vi "Update Custom Device XML.vi"(5 "Template Folder":path, 8 "error in":errorcluster, 10 "Custom Device Name":string, 11 "CDEW_MetaDataObj in":refnum<class "NIVS_CDEW_MetaDataObj.lvclass">) -> (0 "error out":errorcluster, 3 "Custom Device XML Path":path)   [LabVIEW 2026, in "NIVS_CDEW_MetaDataObj.lvclass"]
uses:
  NIVS_CDEW_MetaDataObj.lvclass
  NIVS_CDEW_MetaDataObj.lvclass/NIVS_CDEW_MetaDataObj.ctl
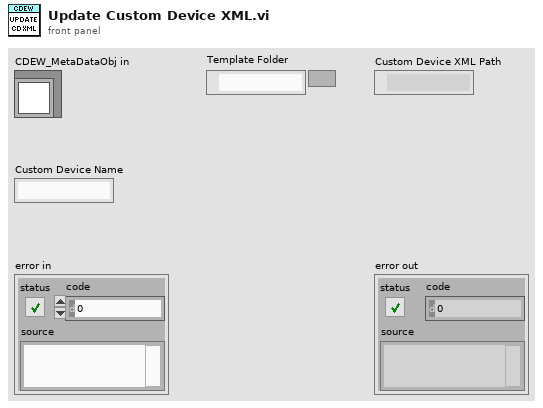
[diagram p1: front panel]
types:
  T1 = typedef "NIVS_CDEW_MetaDataObj.lvclass/Execution Modes.ctl" = enum16{"Inline HW Interface (Inline-Async API)", "Inline HW Interface", "Inline Timing and Sync"}
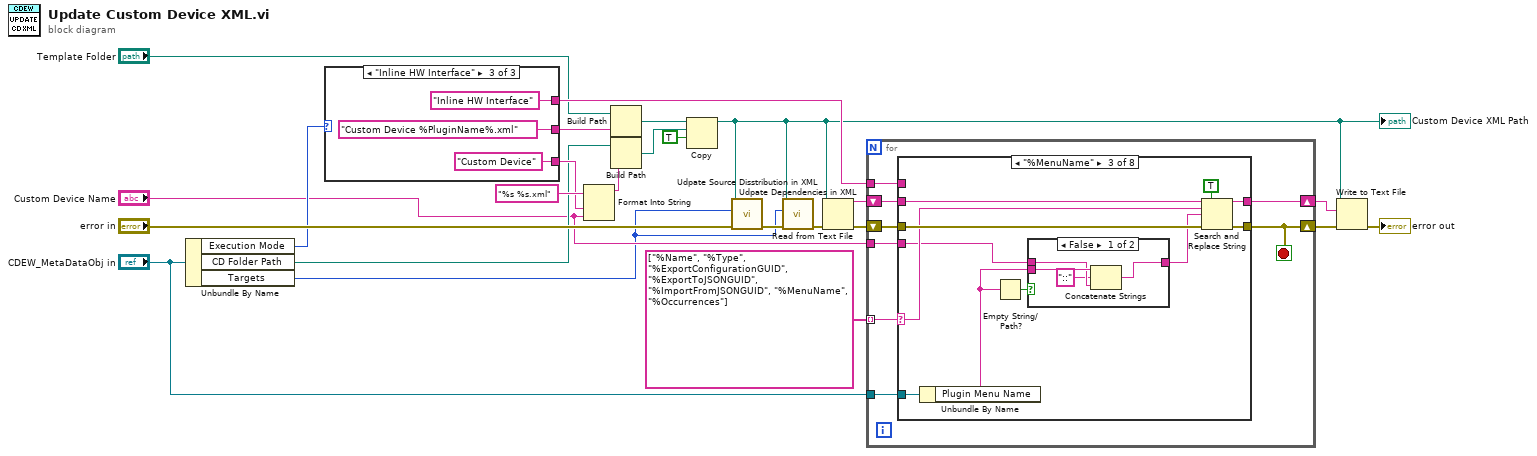
[diagram p0: block diagram]
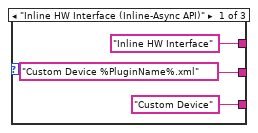
[diagram p2: hidden frame]
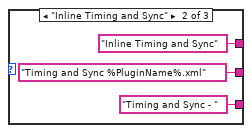
[diagram p3: hidden frame]
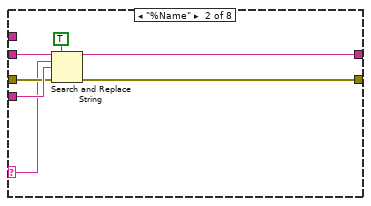
[diagram p5: hidden frame]
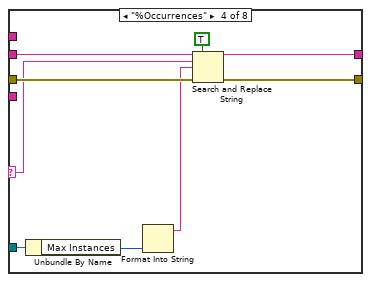
[diagram p7: hidden frame]
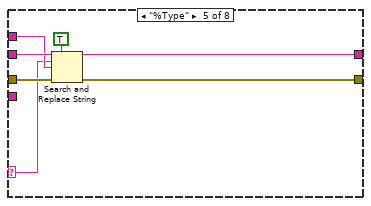
[diagram p8: hidden frame]
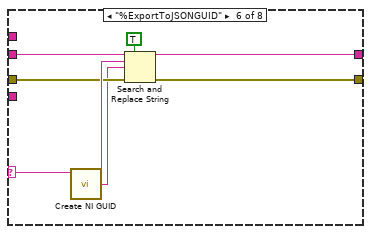
[diagram p9: hidden frame]
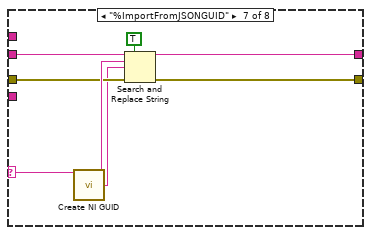
[diagram p10: hidden frame]
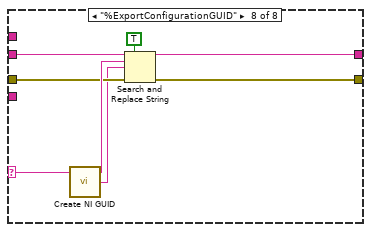
[diagram p11: hidden frame]
diagram:
  n1 = Unbundle By Name("CDEW_MetaDataObj in") -> ("Execution Mode"=w7:T1, "CD Folder Path"=w8:path, "Targets"=w1:enum16{"Linux_x64", "Windows", "Both"})
  n2 = case shown="\"Inline HW Interface\"" w7 {
    tunnel: ["Inline HW Interface" ("Plugin Type") "Inline Timing and Sync" ("Plugin Type") "Inline HW Interface" ("Plugin Type")] -> w18
    tunnel: ["Custom Device %PluginName%.xml" "Timing and Sync %PluginName%.xml" "Custom Device %PluginName%.xml"] -> w16
    tunnel: ["Custom Device" ("Plugin Type") "Timing and Sync - " ("Plugin Type") "Custom Device" ("Plugin Type")] -> w11
    frame "Inline HW Interface (Inline-Async API)" {
    }
    frame "Inline Timing and Sync" {
    }
    frame "Inline HW Interface" {
    }
  }
  n3 = Format Into String(format string="%s %s.xml", w11, "Custom Device Name") -> (resulting string=w10:string)  [unwired: 2 in, 1 out]
  n4 = Build Path(base path="Template Folder", name or relative path=w16) -> (appended path=w15:path)
  n5 = Build Path(base path=w8, name or relative path=w10) -> (appended path=w14:path)
  n6 = Copy(9:TRUE ("overwrite (F)"), 10:w14, 11:w15) -> (3:w2:path)  [unwired: 2 in, 2 out]
  "Custom Device XML Path" <- w2
  n7 = call "Udpate Source Disstribution in XML.vi"("error in"="error in", "Targets"=w1, "XML path"=w2) -> ("error out"=w4:errorcluster)  [unwired: 8 in]
  n8 = call "Udpate Dependencies in XML.vi"("error in"=w4, "Targets"=w1, "XML path"=w2) -> ("error out"=w3:errorcluster)  [unwired: 8 in]
  n9 = Read from Text File(file (use dialog)=w2, error in=w3) -> (text=w23:string, error out=w20:errorcluster)  [unwired: 2 in, 2 out]
  n10 = for {
    tunnel: string[] ["%Name", "%Type", "%ExportConfigurationGUID", "%ExportToJSONGUID", "%ImportFromJSONGUID", "%MenuName", "%Occurrences"] -> [w39] mode=indexing
    shift-right: [w40] -> w22
    shift-left: w23 -> [w41]
    tunnel: "Custom Device Name" -> [w38]
    tunnel: w18 -> [w37]
    shift-right: [w35] -> w19
    shift-left: w20 -> [w36]
    tunnel: "CDEW_MetaDataObj in" -> [w34]
    stop <- w35 stop-if-true
    n11 = case shown="\"%MenuName\"" w39 {
      selector: w39 -> [_ w44 w56 w70 w77 w86 w93 w100]
      tunnel: w41 -> [w43 w50 w61 w75 w82 w89 w96 w103]
      tunnel: [w43 w49 w60 w74 w81 w88 w95 w102] -> w40
      tunnel: w38 -> [_ w48 w54 _ _ _ _ _]
      tunnel: w37 -> [_ _ _ _ w79 _ _ _]
      tunnel: w36 -> [w42 w46 w58 w72 w78 w85 w92 w98]
      tunnel: [w42 w45 w57 w71 w76 w84 w91 w99] -> w35
      tunnel: w34 -> [_ _ w52 w68 _ _ _ _]
      frame Default {
      }
      frame "%Name" {
        n12 = Search and Replace String(replace all?=TRUE ("replace all? (F)"), input string=w50, search string=w44, replace string=w48, error in=w46) -> (result string=w49:string, error out=w45:errorcluster)  [unwired: 3 in, 2 out]
      }
      frame "%MenuName" {
        n13 = Unbundle By Name(w52) -> ("Plugin Menu Name"=w51:string)
        n14 = Empty String/Path?(string/path=w51) -> (empty?=w55:bool)
        n15 = case shown="False" w55 {
          tunnel: [w62 w66] -> w53
          tunnel: w54 -> [w64 w66]
          tunnel: w51 -> [w65 _]
          frame False {
            n16 = Concatenate Strings(w65, "::" ("string"), w64) -> (w62:string)
          }
          frame True {
          }
        }
        n17 = Search and Replace String(replace all?=TRUE ("replace all? (F)"), input string=w61, search string=w56, replace string=w53, error in=w58) -> (result string=w60:string, error out=w57:errorcluster)  [unwired: 3 in, 2 out]
      }
      frame "%Occurrences" {
        n18 = Unbundle By Name(w68) -> ("Max Instances"=w67:i32)
        n19 = Format Into String(w67) -> (resulting string=w69:string)  [unwired: 3 in, 1 out]
        n20 = Search and Replace String(replace all?=TRUE ("replace all? (F)"), input string=w75, search string=w70, replace string=w69, error in=w72) -> (result string=w74:string, error out=w71:errorcluster)  [unwired: 3 in, 2 out]
      }
      frame "%Type" {
        n21 = Search and Replace String(replace all?=TRUE ("replace all? (F)"), input string=w82, search string=w77, replace string=w79, error in=w78) -> (result string=w81:string, error out=w76:errorcluster)  [unwired: 3 in, 2 out]
      }
      frame "%ExportToJSONGUID" {
        n22 = call <vilib>:"Create NI GUID.vi"() -> ("NI GUID"=w83:string)
        n23 = Search and Replace String(replace all?=TRUE ("replace all? (F)"), input string=w89, search string=w86, replace string=w83, error in=w85) -> (result string=w88:string, error out=w84:errorcluster)  [unwired: 3 in, 2 out]
      }
      frame "%ImportFromJSONGUID" {
        n24 = call <vilib>:"Create NI GUID.vi"() -> ("NI GUID"=w90:string)
        n25 = Search and Replace String(replace all?=TRUE ("replace all? (F)"), input string=w96, search string=w93, replace string=w90, error in=w92) -> (result string=w95:string, error out=w91:errorcluster)  [unwired: 3 in, 2 out]
      }
      frame "%ExportConfigurationGUID" {
        n26 = call <vilib>:"Create NI GUID.vi"() -> ("NI GUID"=w97:string)
        n27 = Search and Replace String(replace all?=TRUE ("replace all? (F)"), input string=w103, search string=w100, replace string=w97, error in=w98) -> (result string=w102:string, error out=w99:errorcluster)  [unwired: 3 in, 2 out]
      }
    }
  }
  n28 = Write to Text File(file (use dialog)=w2, text=w22, error in=w19) -> (error out=→"error out":errorcluster)  [unwired: 1 in, 2 out]
